vi "GenerateAnalogWaveformPiezoTraj - ZPiezo_FeedGalvo.vi"(8 "error in (no error)":errorcluster, 11 "SetupInfo_IN":T1={"ConfigParameters_Analog"={"JAI camera fps"=240.0, "Bi-Lateral Galvo xy scan range (V)"=0.7, "Bi-Lateral Galvo xy scan frequency (Hz)"=500, "AOM Blind percent (%)"=0.1, "AOM start blind percent (%) "=70.0, "ROI threshold"=1.0, "AO Sampling rate"=1000000.0}, "ConfigParameters_Digital"={"Steps per volume"=25.0, "Time per volume (s)"=0.4, "OG start layer"=15.0, "Objective Lin Rising Vel (micron/ms）"=1.0, "Image depth (micron)"=200.0, "OG latency (s)"=10.0, "OG repitation"=3.0, "OG end layer"=17.0, "Shock1 duration (s)"=0.001, "Shock2 duration (s)"=0.001, "Shock3 duration (s)"=0.01, "Shock4 duration (s)"=0.01, "Shock5 duration (s)"=0.1, "Shock duration_New"=[]}, "ConfigParameters_Other1"={"Frontal Galvo xy scan range (V)"=0.14, "Frontal Galvo xy scan frequency (Hz)"=500, "PFI 0 digital clock frequency"=500000.0, "Window size for layer index"=0.5, "sCMOS fps"=95.0}, "ConfigParameters_Others2"={"#Trials baseline"=6, "#Trials test"=6, "Time before acq. (s)"=360.0, "Time before test (s)"=600.0, "#Blocks acquisition"=5, "Inter-trial interval baseline (s)"=60.0, "#Trials per acquition block"=6, "Inter-block interval acquisition (s)"=360.0, "Inter-trial interval acquisition (s)"=20.0, "Flash latency (s)"=10.0, "Flash duration (s)"=3.2, "Response duration (s)"=10.0, "MaxTimeEventDetection (s)"=6, "StimType"=enum."Flash", "#MaxEvents"=6}, "ProcessParametersOut"={"stand Z vol Acquisition time (s)"=0.2631578947368421, "stand Z vol Backward time (s)"=0.13684210526315793, "Objective scan volt"=5.0, "Bi-lateral Galvo Z scan volt"=0.1800000180000018, "Frontal Galvo Z scan volt"=0.14940000509752818, "Objective step length (micron)"=8.0, "OG Z volet Linear Dec time (s)"=0.024, "OG Z vol Stim. steps time (s)"=0.031578947368421054, "OG Z vol Linear Acc time (s)"=0.112, "#Vol. of flash"=8, "#Vol. of shock"=1, "#Vol. bef flash"=25, "#Vol. aft flash"=17, "OG Z vol Linear Dec time (s)"=0.112, "OG Z vol time (s)"=0.39073684210526316, "Stack duration"=[0.001, 0.001, 0.01, 0.01, 0.1], "AOM stand. value size"=400000, "Plane indexing length"=0, "#Vol. blank"=0, "#Vol. blank before acq"=0, "#Vol. blank before test"=0, " #Inter-block interval acquisition (Ed-St Vol)"=0}, "WaveformParameters"={"stand Z vol Acquisition samp info"={"Fs"=1000000.0, "#s"=263158.0}, "stand Z vol Backward samp info"={"Fs"=1000000.0, "#s"=136842.0}, "OG Z vol Linear Acc samp info"={"Fs"=1000000.0, "#s"=112000.0}, "OG Z vol Stim. steps samp info"={"Fs"=1000000.0, "#s"=31579.0}, "OG Z volet Linear Dec samp info"={"Fs"=1000000.0, "#s"=24000.0}, "OG Z vol Linear Dec samp info"={"Fs"=1000000.0, "#s"=112000.0}, "OG Z vol samp info"={"Fs"=1000000.0, "#s"=390737.0}, "stand Z vol backforth samp info"={"Fs"=1000000.0, "#s"=400000.0}}, "AnalogWaveform"={"Bi-lateral Galvo Z stand waveform"={"t0"=timestamp(0 s since 1904-01-01), "dt"=1.0, "Y"=[]}, "Frontal Galvo Z stand waveform"={"t0"=timestamp(0 s since 1904-01-01), "dt"=1.0, "Y"=[]}, "Bi-lateral Galvo XY stand waveform"={"t0"=timestamp(0 s since 1904-01-01), "dt"=1.0, "Y"=[]}, "Frontal Galvo XY stand waveform"={"t0"=timestamp(0 s since 1904-01-01), "dt"=1.0, "Y"=[]}, "sCMOS stand waveform"={"t0"=timestamp(0 s since 1904-01-01), "dt"=1.0, "Y"=[]}, "Detection objective stand waveform"={"t0"=timestamp(0 s since 1904-01-01), "dt"=1.0, "Y"=[]}, "AOM stand waveform"={"t0"=timestamp(0 s since 1904-01-01), "dt"=1.0, "Y"=[]}, "PFI 0 clock stand waveform"={"t0"=timestamp(0 s since 1904-01-01), "dt"=1.0, "Y"=[]}, "Bi-lateral Galvo Z OG waveform"={"t0"=timestamp(0 s since 1904-01-01), "dt"=1.0, "Y"=[]}, "Bi-lateral Galvo XY OG waveform"={"t0"=timestamp(0 s since 1904-01-01), "dt"=1.0, "Y"=[]}, "Frontal Galvo Z OG waveform"={"t0"=timestamp(0 s since 1904-01-01), "dt"=1.0, "Y"=[]}, "Frontal Galvo XY OG waveform"={"t0"=timestamp(0 s since 1904-01-01), "dt"=1.0, "Y"=[]}, "sCMOS OG waveform"={"t0"=timestamp(0 s since 1904-01-01), "dt"=1.0, "Y"=[]}, "Detection objective OG waveform"={"t0"=timestamp(0 s since 1904-01-01), "dt"=1.0, "Y"=[]}, "AOM OG waveform"={"t0"=timestamp(0 s since 1904-01-01), "dt"=1.0, "Y"=[]}, "PFI 0 clock OG wavee"={"t0"=timestamp(0 s since 1904-01-01), "dt"=1.0, "Y"=[]}, "sCMOS blank waveform"={"t0"=timestamp(0 s since 1904-01-01), "dt"=1.0, "Y"=[]}, "All analog OG wave"=[], "All analog stand wave"=[], "All analog blank wave"=[], "BufferWaveform_Analog"=[], "Bi-lateral Galvo Z XY"={"t0"=timestamp(0 s since 1904-01-01), "dt"=1.0, "Y"=[]}, "Frontal Galvo Z XY"={"t0"=timestamp(0 s since 1904-01-01), "dt"=1.0, "Y"=[]}, "sCMOS Trigger XY"={"t0"=timestamp(0 s since 1904-01-01), "dt"=1.0, "Y"=[]}, "Detection objective XY"={"t0"=timestamp(0 s since 1904-01-01), "dt"=1.0, "Y"=[]}, "AOM XY"={"t0"=timestamp(0 s since 1904-01-01), "dt"=1.0, "Y"=[]}, "Analog_XY"=[]}, "DigitalWaveform"={"AllDigitalStandWave"=[], "AllDigialEvokedWave"=[], "AllDigialOGWave"=[], "AllDigitalPairWave_1"=[], "AllDigitalPairWave_2"=[], "AllDigitalPairWave_3"=[], "AllDigitalPairWave_4"=[], "AllDigitalPairWave_5"=[], "Plane Indexing"={"t0"=timestamp(0 s since 1904-01-01), "dt"=0.0, "Y"={"transitions"=[], "data"=[]}, "error"={"status"=FALSE, "code"=37421928, "source"=""}}, "Plane indexing P0.5 OG"={"t0"=timestamp(0 s since 1904-01-01), "dt"=0.0, "Y"={"transitions"=[], "data"=[]}, "error"={"status"=FALSE, "code"=37421928, "source"=""}}, "AllDigitalPairWaves"=[], "BufferWaveform_Digital"=[], "AllDigitalBlankWave"=[], "Digial_XY"=[]}, "PhysicalResource"={"PhysicalChannels_AI"="", "PhysicalChannels_AO"="", "PhysicalChannels_DO"="", "Task_AnalogOutput"="", "Task_DigitalOutput"="", "Task_AnalogInput"=""}, "ControlsRef"={"Mode_1"=refnum, "EventDetectionMode"=refnum, "Mode_2A"=refnum, "StimulationMode"=refnum, "Mode_2B"=refnum, "ErrorMeg"=refnum}} {"ConfigParameters_Other1"."Frontal Galvo xy scan frequency (Hz)" min=500 max=500; "ConfigParameters_Other1"."Frontal Galvo xy scan range (V)" min=0.0 max=1.5; "ConfigParameters_Analog"."AOM start blind percent (%)" min=10.0 max=90.0; "ConfigParameters_Analog"."AOM Blind percent (%)" min=0.1 max=100.0; "ConfigParameters_Analog"."Bi-Lateral Galvo xy scan frequency (Hz)" min=500 max=500; "ConfigParameters_Analog"."Bi-Lateral Galvo xy scan range (V)" min=0.0 max=1.5}) -> (0 "error out":errorcluster, 3 "SetupInfo_OUT":T1={"ConfigParameters_Analog"={"JAI camera fps"=240.0, "Bi-Lateral Galvo xy scan range (V)"=0.7, "Bi-Lateral Galvo xy scan frequency (Hz)"=500, "AOM Blind percent (%)"=0.1, "AOM start blind percent (%) "=70.0, "ROI threshold"=1.0, "AO Sampling rate"=1000000.0}, "ConfigParameters_Digital"={"Steps per volume"=25.0, "Time per volume (s)"=0.4, "OG start layer"=15.0, "Objective Lin Rising Vel (micron/ms）"=1.0, "Image depth (micron)"=200.0, "OG latency (s)"=10.0, "OG repitation"=3.0, "OG end layer"=17.0, "Shock1 duration (s)"=0.001, "Shock2 duration (s)"=0.001, "Shock3 duration (s)"=0.01, "Shock4 duration (s)"=0.01, "Shock5 duration (s)"=0.1, "Shock duration_New"=[]}, "ConfigParameters_Other1"={"Frontal Galvo xy scan range (V)"=0.14, "Frontal Galvo xy scan frequency (Hz)"=500, "PFI 0 digital clock frequency"=500000.0, "Window size for layer index"=0.5, "sCMOS fps"=95.0}, "ConfigParameters_Others2"={"#Trials baseline"=6, "#Trials test"=6, "Time before acq. (s)"=360.0, "Time before test (s)"=600.0, "#Blocks acquisition"=5, "Inter-trial interval baseline (s)"=60.0, "#Trials per acquition block"=6, "Inter-block interval acquisition (s)"=360.0, "Inter-trial interval acquisition (s)"=20.0, "Flash latency (s)"=10.0, "Flash duration (s)"=3.2, "Response duration (s)"=10.0, "MaxTimeEventDetection (s)"=6, "StimType"=enum."Flash", "#MaxEvents"=6}, "ProcessParametersOut"={"stand Z vol Acquisition time (s)"=0.2631578947368421, "stand Z vol Backward time (s)"=0.13684210526315793, "Objective scan volt"=5.0, "Bi-lateral Galvo Z scan volt"=0.1800000180000018, "Frontal Galvo Z scan volt"=0.14940000509752818, "Objective step length (micron)"=8.0, "OG Z volet Linear Dec time (s)"=0.024, "OG Z vol Stim. steps time (s)"=0.031578947368421054, "OG Z vol Linear Acc time (s)"=0.112, "#Vol. of flash"=8, "#Vol. of shock"=1, "#Vol. bef flash"=25, "#Vol. aft flash"=17, "OG Z vol Linear Dec time (s)"=0.112, "OG Z vol time (s)"=0.39073684210526316, "Stack duration"=[0.001, 0.001, 0.01, 0.01, 0.1], "AOM stand. value size"=400000, "Plane indexing length"=0, "#Vol. blank"=0, "#Vol. blank before acq"=0, "#Vol. blank before test"=0, " #Inter-block interval acquisition (Ed-St Vol)"=0}, "WaveformParameters"={"stand Z vol Acquisition samp info"={"Fs"=1000000.0, "#s"=263158.0}, "stand Z vol Backward samp info"={"Fs"=1000000.0, "#s"=136842.0}, "OG Z vol Linear Acc samp info"={"Fs"=1000000.0, "#s"=112000.0}, "OG Z vol Stim. steps samp info"={"Fs"=1000000.0, "#s"=31579.0}, "OG Z volet Linear Dec samp info"={"Fs"=1000000.0, "#s"=24000.0}, "OG Z vol Linear Dec samp info"={"Fs"=1000000.0, "#s"=112000.0}, "OG Z vol samp info"={"Fs"=1000000.0, "#s"=390737.0}, "stand Z vol backforth samp info"={"Fs"=1000000.0, "#s"=400000.0}}, "AnalogWaveform"={"Bi-lateral Galvo Z stand waveform"={"t0"=timestamp(0 s since 1904-01-01), "dt"=1.0, "Y"=[]}, "Frontal Galvo Z stand waveform"={"t0"=timestamp(0 s since 1904-01-01), "dt"=1.0, "Y"=[]}, "Bi-lateral Galvo XY stand waveform"={"t0"=timestamp(0 s since 1904-01-01), "dt"=1.0, "Y"=[]}, "Frontal Galvo XY stand waveform"={"t0"=timestamp(0 s since 1904-01-01), "dt"=1.0, "Y"=[]}, "sCMOS stand waveform"={"t0"=timestamp(0 s since 1904-01-01), "dt"=1.0, "Y"=[]}, "Detection objective stand waveform"={"t0"=timestamp(0 s since 1904-01-01), "dt"=1.0, "Y"=[]}, "AOM stand waveform"={"t0"=timestamp(0 s since 1904-01-01), "dt"=1.0, "Y"=[]}, "PFI 0 clock stand waveform"={"t0"=timestamp(0 s since 1904-01-01), "dt"=1.0, "Y"=[]}, "Bi-lateral Galvo Z OG waveform"={"t0"=timestamp(0 s since 1904-01-01), "dt"=1.0, "Y"=[]}, "Bi-lateral Galvo XY OG waveform"={"t0"=timestamp(0 s since 1904-01-01), "dt"=1.0, "Y"=[]}, "Frontal Galvo Z OG waveform"={"t0"=timestamp(0 s since 1904-01-01), "dt"=1.0, "Y"=[]}, "Frontal Galvo XY OG waveform"={"t0"=timestamp(0 s since 1904-01-01), "dt"=1.0, "Y"=[]}, "sCMOS OG waveform"={"t0"=timestamp(0 s since 1904-01-01), "dt"=1.0, "Y"=[]}, "Detection objective OG waveform"={"t0"=timestamp(0 s since 1904-01-01), "dt"=1.0, "Y"=[]}, "AOM OG waveform"={"t0"=timestamp(0 s since 1904-01-01), "dt"=1.0, "Y"=[]}, "PFI 0 clock OG wavee"={"t0"=timestamp(0 s since 1904-01-01), "dt"=1.0, "Y"=[]}, "sCMOS blank waveform"={"t0"=timestamp(0 s since 1904-01-01), "dt"=1.0, "Y"=[]}, "All analog OG wave"=[], "All analog stand wave"=[], "All analog blank wave"=[], "BufferWaveform_Analog"=[], "Bi-lateral Galvo Z XY"={"t0"=timestamp(0 s since 1904-01-01), "dt"=1.0, "Y"=[]}, "Frontal Galvo Z XY"={"t0"=timestamp(0 s since 1904-01-01), "dt"=1.0, "Y"=[]}, "sCMOS Trigger XY"={"t0"=timestamp(0 s since 1904-01-01), "dt"=1.0, "Y"=[]}, "Detection objective XY"={"t0"=timestamp(0 s since 1904-01-01), "dt"=1.0, "Y"=[]}, "AOM XY"={"t0"=timestamp(0 s since 1904-01-01), "dt"=1.0, "Y"=[]}, "Analog_XY"=[]}, "DigitalWaveform"={"AllDigitalStandWave"=[], "AllDigialEvokedWave"=[], "AllDigialOGWave"=[], "AllDigitalPairWave_1"=[], "AllDigitalPairWave_2"=[], "AllDigitalPairWave_3"=[], "AllDigitalPairWave_4"=[], "AllDigitalPairWave_5"=[], "Plane Indexing"={"t0"=timestamp(0 s since 1904-01-01), "dt"=0.0, "Y"={"transitions"=[], "data"=[]}, "error"={"status"=FALSE, "code"=37421928, "source"=""}}, "Plane indexing P0.5 OG"={"t0"=timestamp(0 s since 1904-01-01), "dt"=0.0, "Y"={"transitions"=[], "data"=[]}, "error"={"status"=FALSE, "code"=37421928, "source"=""}}, "AllDigitalPairWaves"=[], "BufferWaveform_Digital"=[], "AllDigitalBlankWave"=[], "Digial_XY"=[]}, "PhysicalResource"={"PhysicalChannels_AI"="", "PhysicalChannels_AO"="", "PhysicalChannels_DO"="", "Task_AnalogOutput"="", "Task_DigitalOutput"="", "Task_AnalogInput"=""}, "ControlsRef"={"Mode_1"=refnum, "EventDetectionMode"=refnum, "Mode_2A"=refnum, "StimulationMode"=refnum, "Mode_2B"=refnum, "ErrorMeg"=refnum}} {"ConfigParameters_Other1"."Frontal Galvo xy scan frequency (Hz)" min=500 max=500; "ConfigParameters_Other1"."Frontal Galvo xy scan range (V)" min=0.0 max=1.5; "ConfigParameters_Analog"."AOM start blind percent (%)" min=10.0 max=90.0; "ConfigParameters_Analog"."AOM Blind percent (%)" min=0.1 max=100.0; "ConfigParameters_Analog"."Bi-Lateral Galvo xy scan frequency (Hz)" min=500 max=500; "ConfigParameters_Analog"."Bi-Lateral Galvo xy scan range (V)" min=0.0 max=1.5})   [LabVIEW 2018]
uses:
  SetupInfo.ctl
  ConfigParameters_Analog.ctl
  ConfigParameters_Digital.ctl
  ConfigParameters_Others1.ctl
  ConfigParameters_Others2.ctl
  ProcessParametersOut.ctl
  WaveformParameters.ctl
  AnalogWaveform.ctl
  DigitalWaveform.ctl
  PhysicalResource.ctl
  ControlsRef.ctl
  <vilib>/Waveform/WDTOps.llb/WDT Append Waveforms DBL.vi
  <vilib>/measure/NI_MABase.lvlib
panel:
  in  "FileSamplingRate":dbl=1000.0
  in  "PiezoTrajectoryPath":path=path "D:/APP/LightSheetController_Ver8 obl/VISource/Waveform/piezo_In_Out.txt"
  out "AOM stand. value size":i32=400000
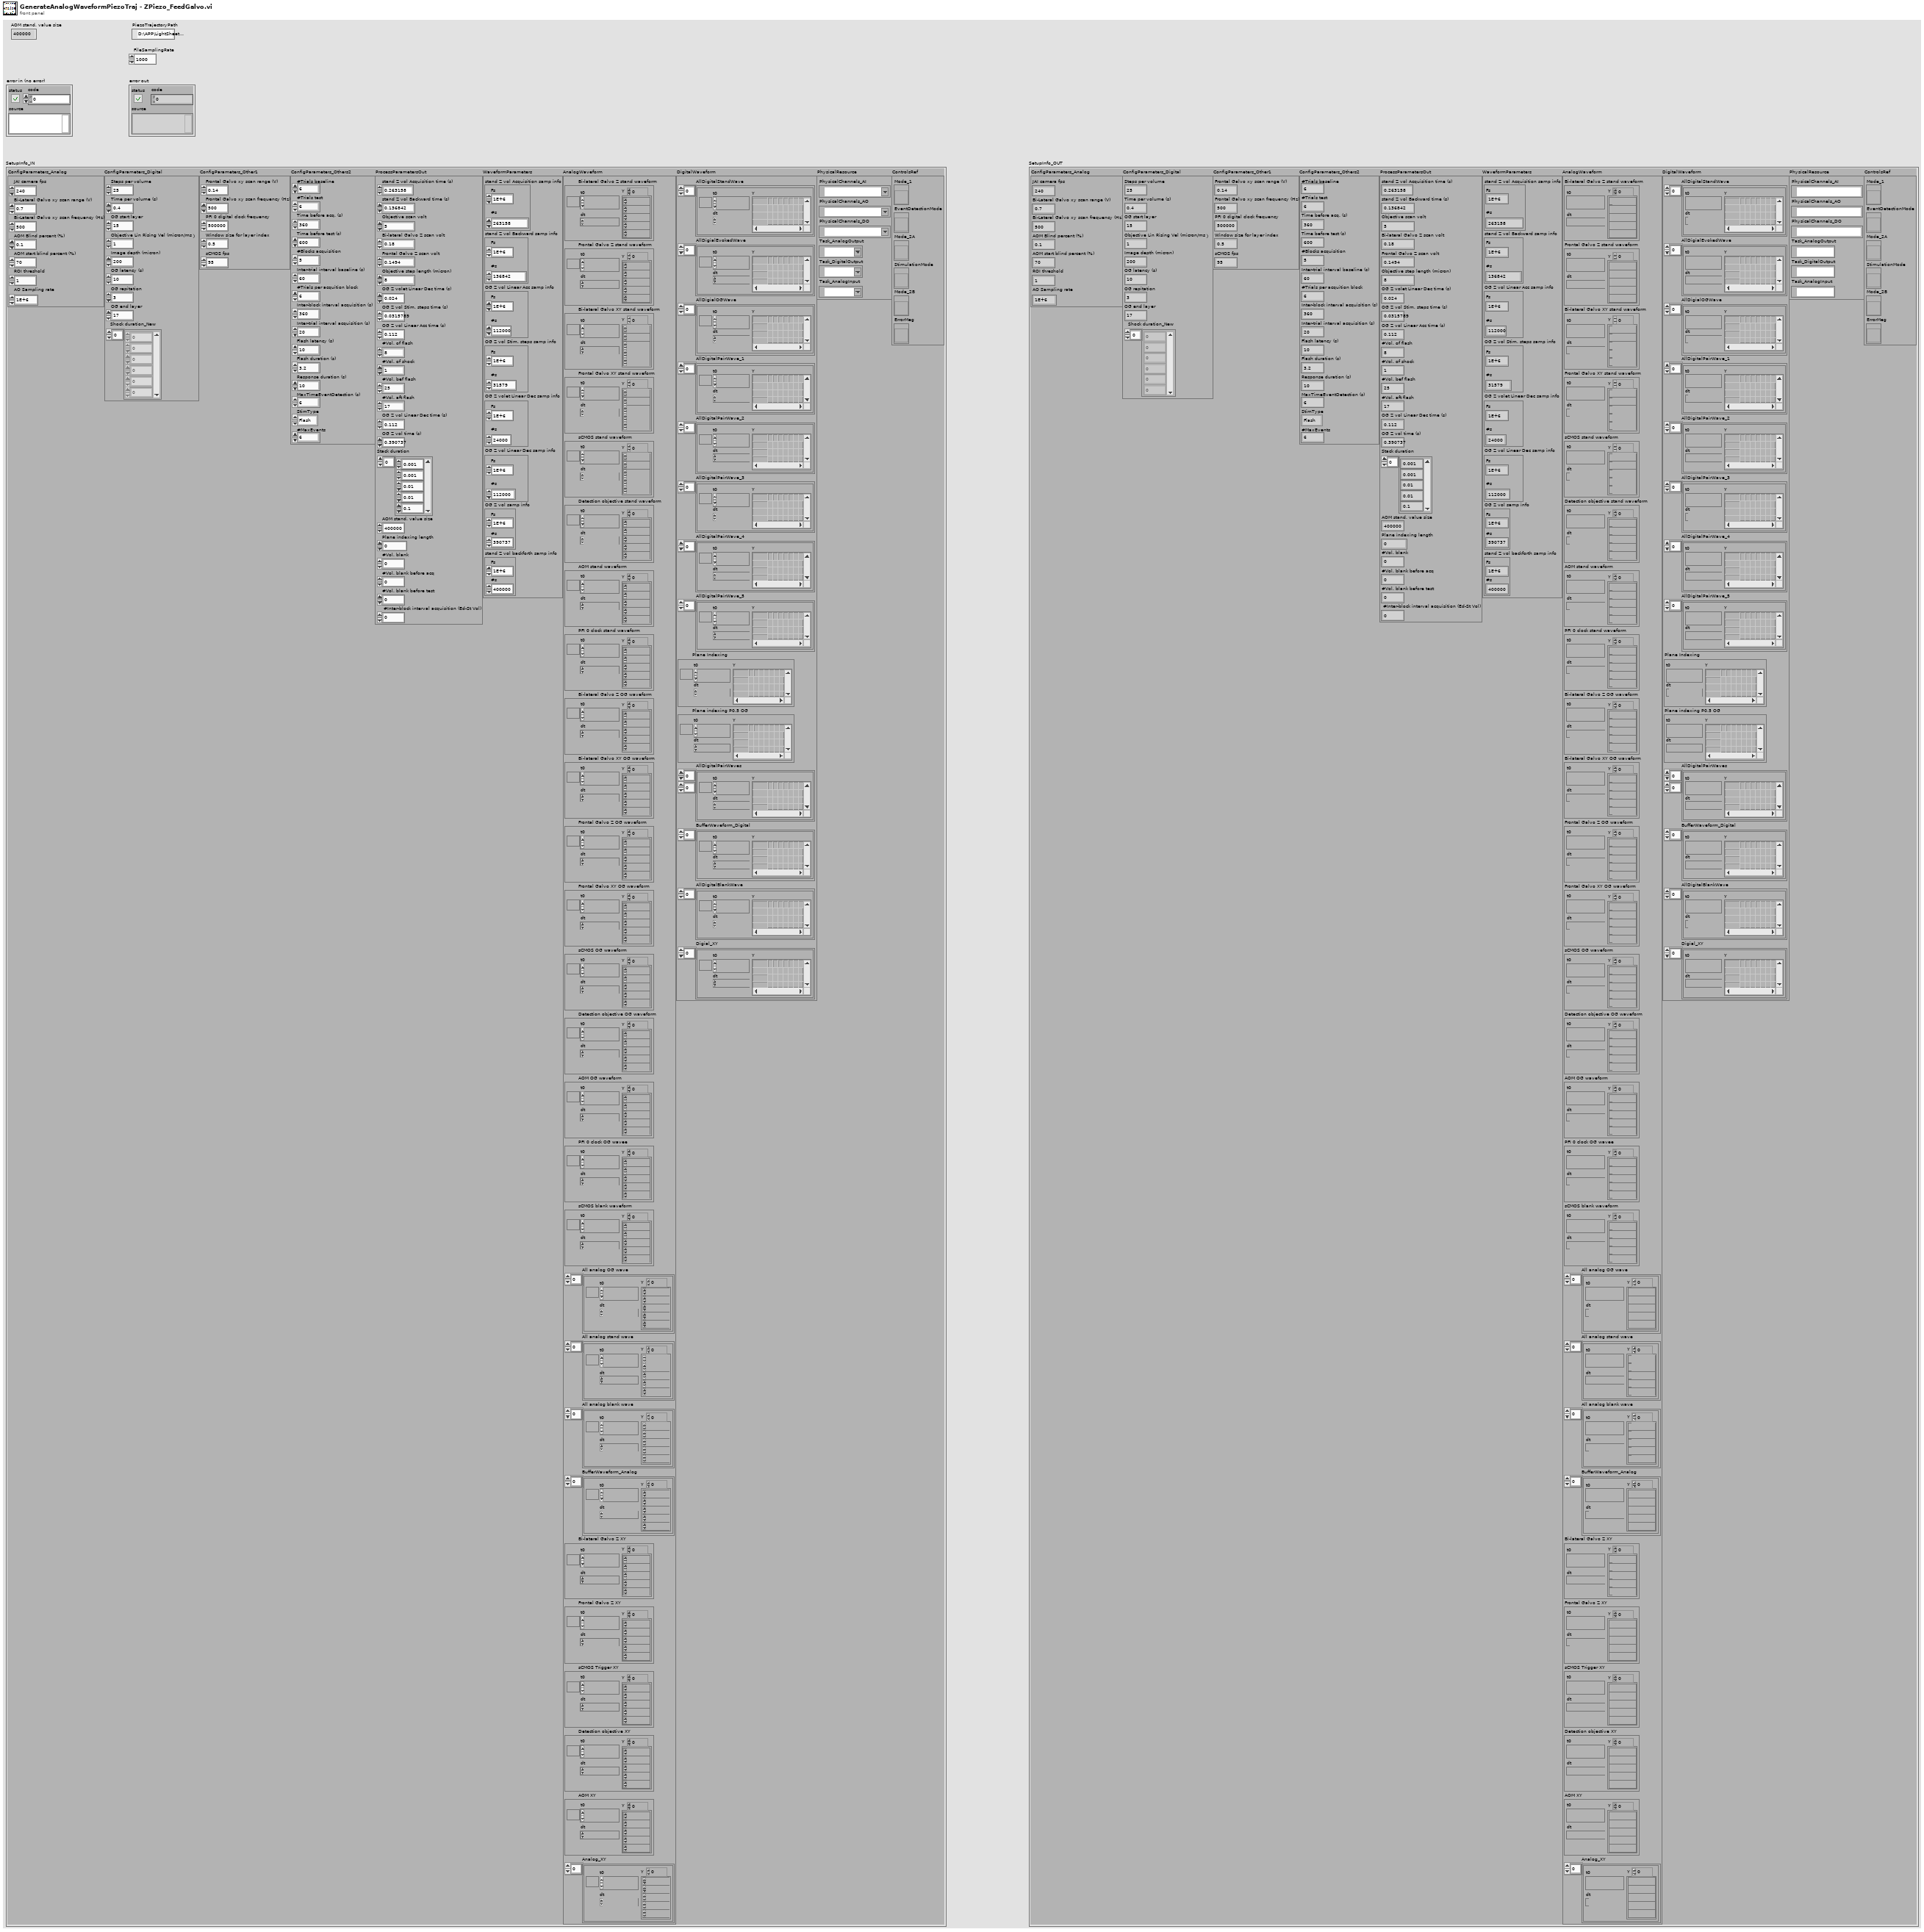
[diagram p1: front panel]
types:
  T1 = typedef "SetupInfo.ctl" = cluster{"ConfigParameters_Analog":T2, "ConfigParameters_Digital":T3, "ConfigParameters_Other1":T4, "ConfigParameters_Others2":T5, "ProcessParametersOut":T6, "WaveformParameters":T7, "AnalogWaveform":T8, "DigitalWaveform":T9, "PhysicalResource":T10, "ControlsRef":T11}
  T2 = typedef "ConfigParameters_Analog.ctl" = cluster{"JAI camera fps":dbl, "Bi-Lateral Galvo xy scan range (V)":dbl, "Bi-Lateral Galvo xy scan frequency (Hz)":i16, "AOM Blind percent (%)":dbl, "AOM start blind percent (%) ":dbl, "ROI threshold":dbl, "AO Sampling rate":dbl}
  T3 = typedef "ConfigParameters_Digital.ctl" = cluster{"Steps per volume":dbl, "Time per volume (s)":dbl, "OG start layer":dbl, "Objective Lin Rising Vel (micron/ms）":dbl, "Image depth (micron)":dbl, "OG latency (s)":dbl, "OG repitation":dbl, "OG end layer":dbl, "Shock1 duration (s)":dbl, "Shock2 duration (s)":dbl, "Shock3 duration (s)":dbl, "Shock4 duration (s)":dbl, "Shock5 duration (s)":dbl, "Shock duration_New":dbl[]}
  T4 = typedef "ConfigParameters_Others1.ctl" = cluster{"Frontal Galvo xy scan range (V)":dbl, "Frontal Galvo xy scan frequency (Hz)":i16, "PFI 0 digital clock frequency":dbl, "Window size for layer index":dbl, "sCMOS fps":dbl}
  T5 = typedef "ConfigParameters_Others2.ctl" = cluster{"#Trials baseline":i32, "#Trials test":i32, "Time before acq. (s)":dbl, "Time before test (s)":dbl, "#Blocks acquisition":i32, "Inter-trial interval baseline (s)":dbl, "#Trials per acquition block":i32, "Inter-block interval acquisition (s)":dbl, "Inter-trial interval acquisition (s)":dbl, "Flash latency (s)":dbl, "Flash duration (s)":dbl, "Response duration (s)":dbl, "MaxTimeEventDetection (s)":i32, "StimType":enum16{"Flash", "OG"}, "#MaxEvents":i32}
  T6 = typedef "ProcessParametersOut.ctl" = cluster{"stand Z vol Acquisition time (s)":dbl, "stand Z vol Backward time (s)":dbl, "Objective scan volt":dbl, "Bi-lateral Galvo Z scan volt":dbl, "Frontal Galvo Z scan volt":dbl, "Objective step length (micron)":dbl, "OG Z volet Linear Dec time (s)":dbl, "OG Z vol Stim. steps time (s)":dbl, "OG Z vol Linear Acc time (s)":dbl, "#Vol. of flash":i32, "#Vol. of shock":i32, "#Vol. bef flash":i32, "#Vol. aft flash":i32, "OG Z vol Linear Dec time (s)":dbl, "OG Z vol time (s)":dbl, "Stack duration":dbl[], "AOM stand. value size":i32, "Plane indexing length":i32, "#Vol. blank":i32, "#Vol. blank before acq":i32, "#Vol. blank before test":i32, " #Inter-block interval acquisition (Ed-St Vol)":i32}
  T7 = typedef "WaveformParameters.ctl" = cluster{"stand Z vol Acquisition samp info":cluster{"Fs":dbl, "#s":dbl}, "stand Z vol Backward samp info":cluster{"Fs":dbl, "#s":dbl}, "OG Z vol Linear Acc samp info":cluster{"Fs":dbl, "#s":dbl}, "OG Z vol Stim. steps samp info":cluster{"Fs":dbl, "#s":dbl}, "OG Z volet Linear Dec samp info":cluster{"Fs":dbl, "#s":dbl}, "OG Z vol Linear Dec samp info":cluster{"Fs":dbl, "#s":dbl}, "OG Z vol samp info":cluster{"Fs":dbl, "#s":dbl}, "stand Z vol backforth samp info":cluster{"Fs":dbl, "#s":dbl}}
  T8 = typedef "AnalogWaveform.ctl" = cluster{"Bi-lateral Galvo Z stand waveform":waveform(dbl), "Frontal Galvo Z stand waveform":waveform(dbl), "Bi-lateral Galvo XY stand waveform":waveform(dbl), "Frontal Galvo XY stand waveform":waveform(dbl), "sCMOS stand waveform":waveform(dbl), "Detection objective stand waveform":waveform(dbl), "AOM stand waveform":waveform(dbl), "PFI 0 clock stand waveform":waveform(dbl), "Bi-lateral Galvo Z OG waveform":waveform(dbl), "Bi-lateral Galvo XY OG waveform":waveform(dbl), "Frontal Galvo Z OG waveform":waveform(dbl), "Frontal Galvo XY OG waveform":waveform(dbl), "sCMOS OG waveform":waveform(dbl), "Detection objective OG waveform":waveform(dbl), "AOM OG waveform":waveform(dbl), "PFI 0 clock OG wavee":waveform(dbl), "sCMOS blank waveform":waveform(dbl), "All analog OG wave":waveform(dbl)[], "All analog stand wave":waveform(dbl)[], "All analog blank wave":waveform(dbl)[], "BufferWaveform_Analog":waveform(dbl)[], "Bi-lateral Galvo Z XY":waveform(dbl), "Frontal Galvo Z XY":waveform(dbl), "sCMOS Trigger XY":waveform(dbl), "Detection objective XY":waveform(dbl), "AOM XY":waveform(dbl), "Analog_XY":waveform(dbl)[]}
  T9 = typedef "DigitalWaveform.ctl" = cluster{"AllDigitalStandWave":digitalwaveform[], "AllDigialEvokedWave":digitalwaveform[], "AllDigialOGWave":digitalwaveform[], "AllDigitalPairWave_1":digitalwaveform[], "AllDigitalPairWave_2":digitalwaveform[], "AllDigitalPairWave_3":digitalwaveform[], "AllDigitalPairWave_4":digitalwaveform[], "AllDigitalPairWave_5":digitalwaveform[], "Plane Indexing":digitalwaveform, "Plane indexing P0.5 OG":digitalwaveform, "AllDigitalPairWaves":digitalwaveform[][], "BufferWaveform_Digital":digitalwaveform[], "AllDigitalBlankWave":digitalwaveform[], "Digial_XY":digitalwaveform[]}
  T10 = typedef "PhysicalResource.ctl" = cluster{"PhysicalChannels_AI":tag, "PhysicalChannels_AO":tag, "PhysicalChannels_DO":tag, "Task_AnalogOutput":refnum<k21>, "Task_DigitalOutput":refnum<k21>, "Task_AnalogInput":refnum<k21>}
  T11 = typedef "ControlsRef.ctl" = cluster{"Mode_1":refnum<vi>, "EventDetectionMode":refnum<vi>, "Mode_2A":refnum<vi>, "StimulationMode":refnum<vi>, "Mode_2B":refnum<vi>, "ErrorMeg":refnum<vi>}
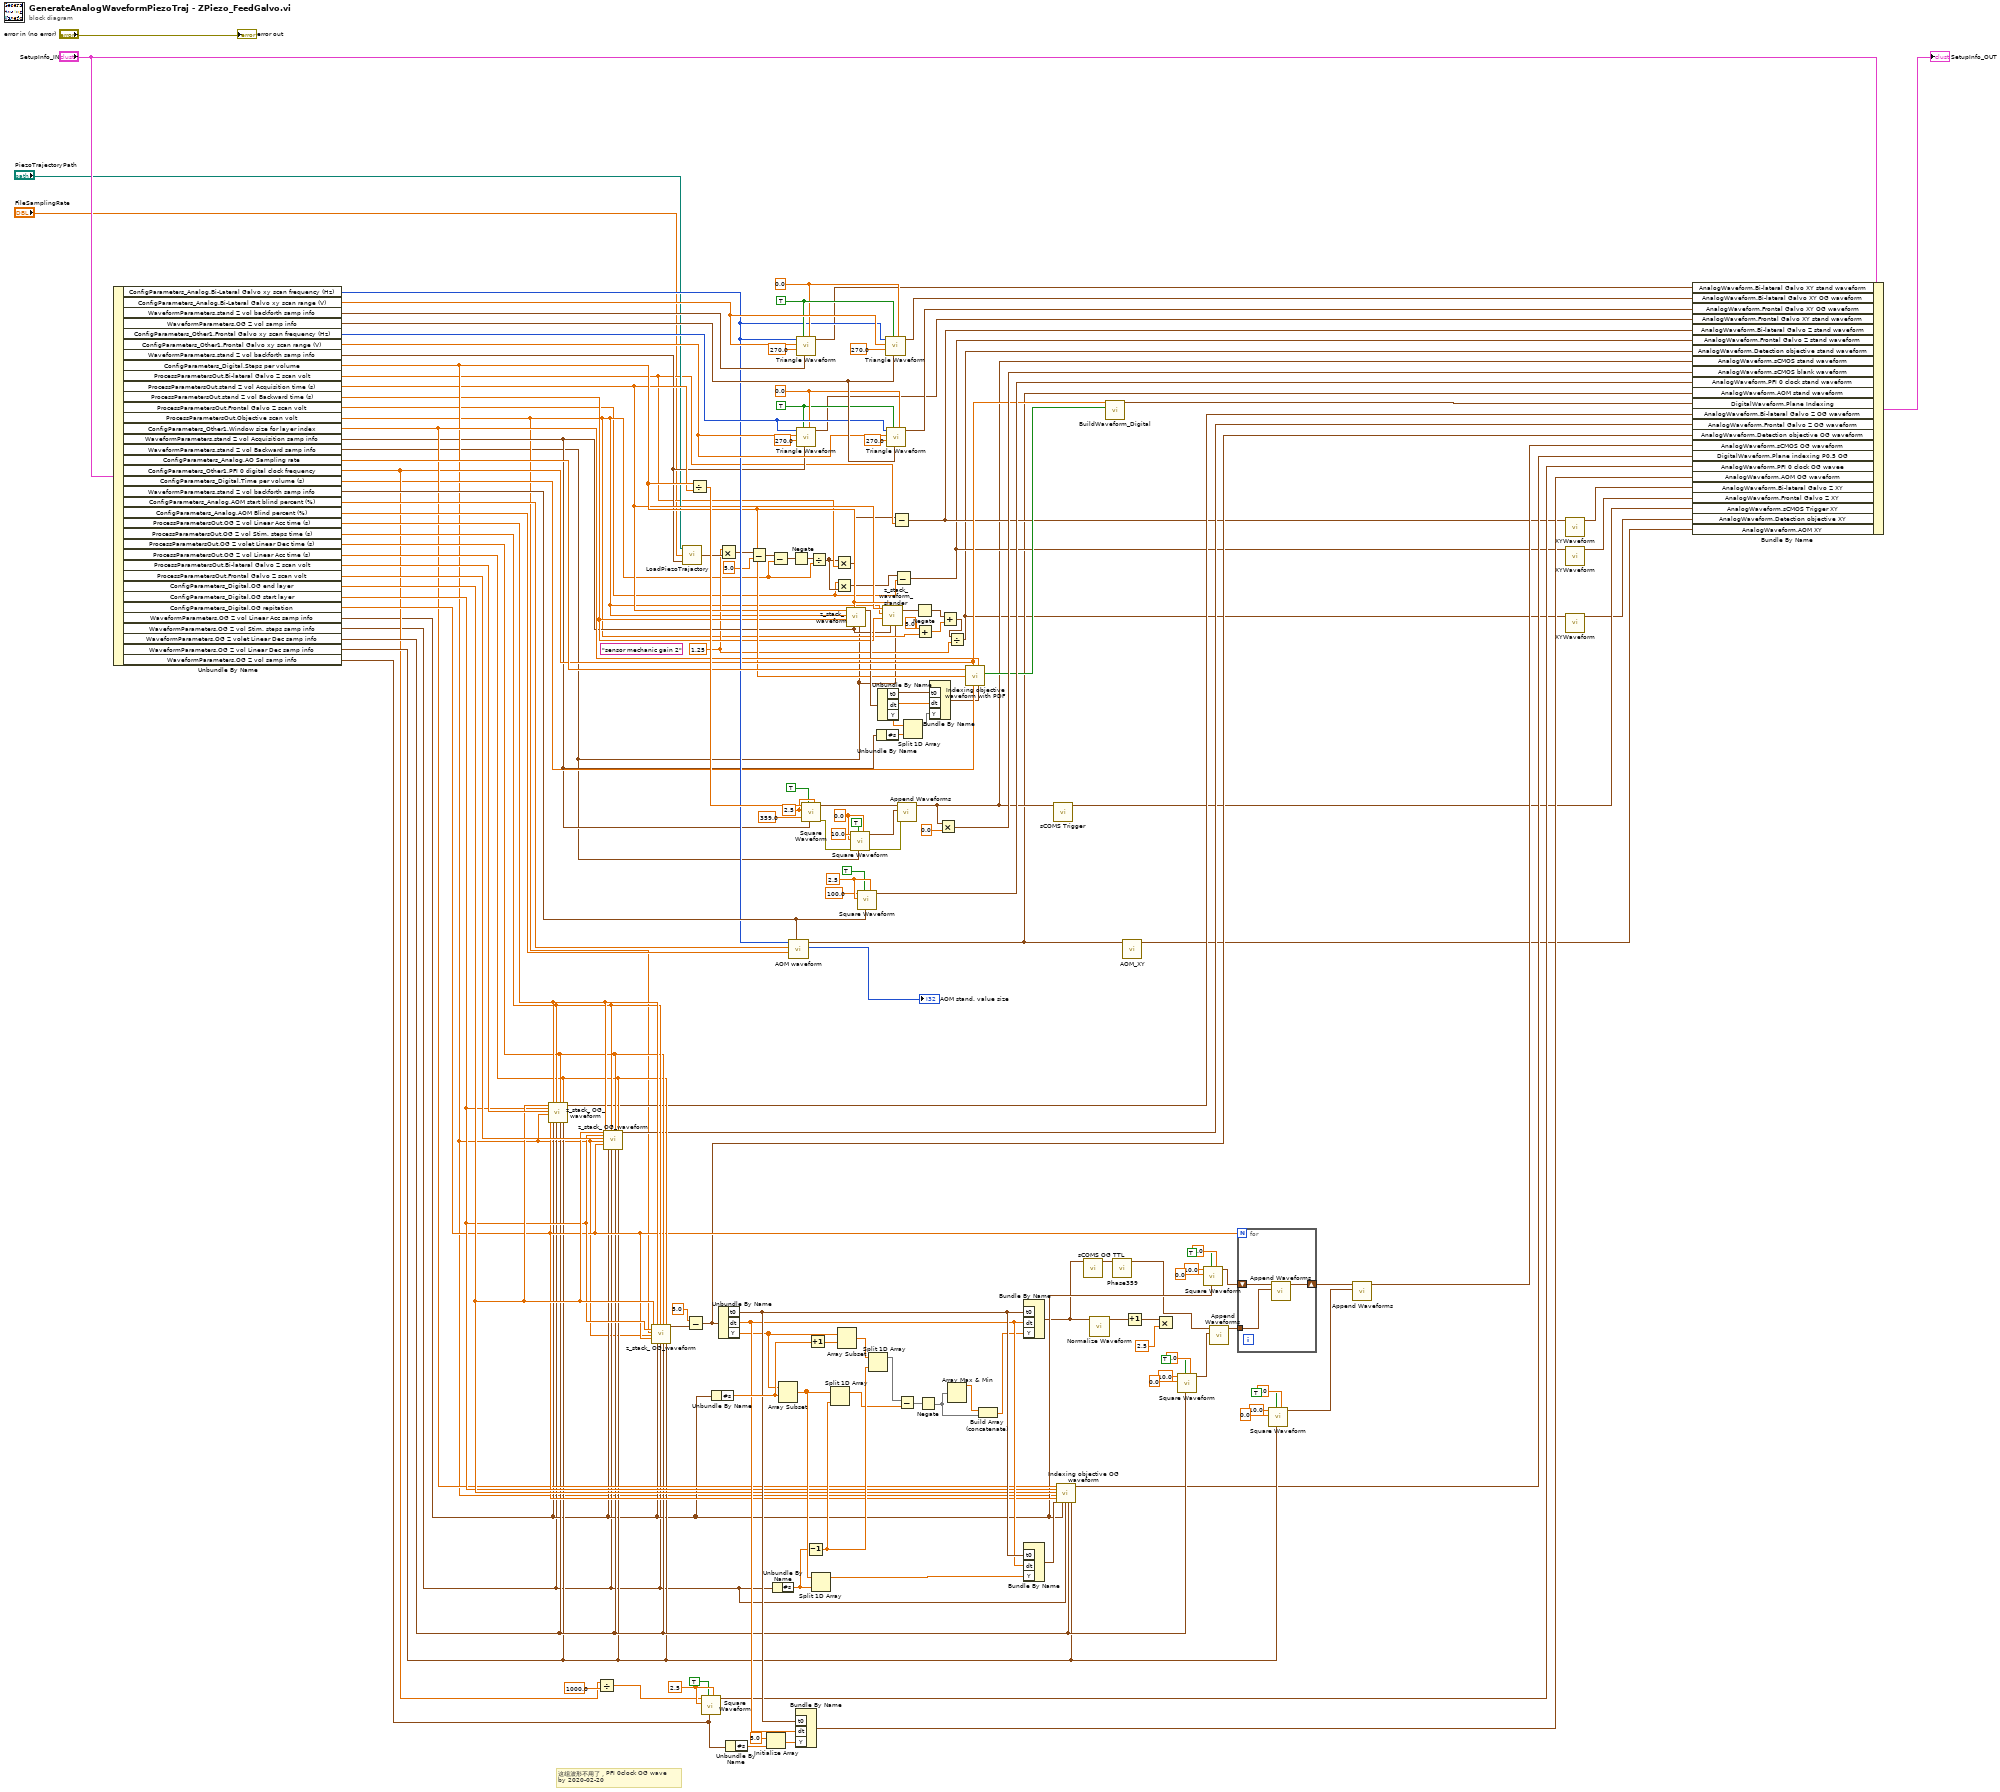
[diagram p0: block diagram]
diagram:
  (unwired) "sensor mechanic gain 2"
  w15 = 1.25
  w91 = 2.5
  w136 = 2.5 ("offset")
  w143 = 0.0 ("offset")
  w147 = 2.5 ("amplitude")
  w122 = TRUE ("reset signal")
  w130 = TRUE ("reset signal")
  w129 = 0.0 ("offset")
  w123 = 0.0 ("offset")
  # "这组波形不用了，PFI 0clock OG wave\nby 2020-02-20"
  n1 = Unbundle By Name("SetupInfo_IN") -> ("ConfigParameters_Analog.Bi-Lateral Galvo xy scan frequency (Hz)"=w118:i16, "ConfigParameters_Analog.Bi-Lateral Galvo xy scan range (V)"=w132:dbl, "WaveformParameters.stand Z vol backforth samp info"=w131:cluster{"Fs":dbl, "#s":dbl}, "WaveformParameters.OG Z vol samp info"=w127:cluster{"Fs":dbl, "#s":dbl}, "ConfigParameters_Other1.Frontal Galvo xy scan frequency (Hz)"=w126:i16, "ConfigParameters_Other1.Frontal Galvo xy scan range (V)"=w125:dbl, "WaveformParameters.stand Z vol backforth samp info"=w18:cluster{"Fs":dbl, "#s":dbl}, "ConfigParameters_Digital.Steps per volume"=w24:dbl, "ProcessParametersOut.Bi-lateral Galvo Z scan volt"=w7:dbl, "ProcessParametersOut.stand Z vol Acquisition time (s)"=w23:dbl, "ProcessParametersOut.stand Z vol Backward time (s)"=w22:dbl, "ProcessParametersOut.Frontal Galvo Z scan volt"=w4:dbl, "ProcessParametersOut.Objective scan volt"=w8:dbl, "ConfigParameters_Other1.Window size for layer index"=w75:dbl, "WaveformParameters.stand Z vol Acquisition samp info"=w21:cluster{"Fs":dbl, "#s":dbl}, "WaveformParameters.stand Z vol Backward samp info"=w2:cluster{"Fs":dbl, "#s":dbl}, "ConfigParameters_Analog.AO Sampling rate"=w120:dbl, "ConfigParameters_Other1.PFI 0 digital clock frequency"=w59:dbl, "ConfigParameters_Digital.Time per volume (s)"=w58:dbl, "WaveformParameters.stand Z vol backforth samp info"=w119:cluster{"Fs":dbl, "#s":dbl}, "ConfigParameters_Analog.AOM start blind percent (%)"=w117:dbl, "ConfigParameters_Analog.AOM Blind percent (%)"=w116:dbl, "ProcessParametersOut.OG Z vol Linear Acc time (s)"=w84:dbl, "ProcessParametersOut.OG Z vol Stim. steps time (s)"=w83:dbl, "ProcessParametersOut.OG Z volet Linear Dec time (s)"=w82:dbl, "ProcessParametersOut.OG Z vol Linear Acc time (s)"=w81:dbl, "ProcessParametersOut.Bi-lateral Galvo Z scan volt"=w80:dbl, "ProcessParametersOut.Frontal Galvo Z scan volt"=w79:dbl, "ConfigParameters_Digital.OG end layer"=w78:dbl, "ConfigParameters_Digital.OG start layer"=w77:dbl, "ConfigParameters_Digital.OG repitation"=w76:dbl, "WaveformParameters.OG Z vol Linear Acc samp info"=w41:cluster{"Fs":dbl, "#s":dbl}, "WaveformParameters.OG Z vol Stim. steps samp info"=w40:cluster{"Fs":dbl, "#s":dbl}, "WaveformParameters.OG Z volet Linear Dec samp info"=w74:cluster{"Fs":dbl, "#s":dbl}, "WaveformParameters.OG Z vol Linear Dec samp info"=w73:cluster{"Fs":dbl, "#s":dbl}, "WaveformParameters.OG Z vol samp info"=w72:cluster{"Fs":dbl, "#s":dbl})
  n2 = call "z_stack_ OG_waveform.vi"("OG end layer"=w78, "OG start layer"=w77, "SPECIFIC scan volt"=w80, "Steps per volume"=w24, "OG repitation"=w76, "Objective线性加速时间"=w84, "OG Z stack 线性加速 采样信息"=w41, "Objective 刺激steps 时间（s）"=w83, "OG Z stack 刺激steps 采样信息"=w40, "Objective volet 线性减速 时间（s）"=w82, "OG Z volet 线性减速 采样信息"=w74, "Objective线性减速时间"=w81, "OG Z stack 线性减速 采样信息"=w73) -> ("waveform out"=w62:waveform(dbl))  [unwired: 2 in, 4 out]
  n3 = Divide(x=w59, y=1000.0) -> (x/y=w65:dbl)
  n4 = call "z_stack_ OG_waveform.vi"("OG end layer"=w78, "OG start layer"=w77, "SPECIFIC scan volt"=w79, "Steps per volume"=w24, "OG repitation"=w76, "Objective线性加速时间"=w84, "OG Z stack 线性加速 采样信息"=w41, "Objective 刺激steps 时间（s）"=w83, "OG Z stack 刺激steps 采样信息"=w40, "Objective volet 线性减速 时间（s）"=w82, "OG Z volet 线性减速 采样信息"=w74, "Objective线性减速时间"=w81, "OG Z stack 线性减速 采样信息"=w73) -> ("waveform out"=w61:waveform(dbl))  [unwired: 2 in, 4 out]
  n5 = call "z_stack_ OG_waveform.vi"("OG end layer"=w78, "OG start layer"=w77, "SPECIFIC scan volt"=w8, "Steps per volume"=w24, "OG repitation"=w76, "Objective线性加速时间"=w84, "OG Z stack 线性加速 采样信息"=w41, "Objective 刺激steps 时间（s）"=w83, "OG Z stack 刺激steps 采样信息"=w40, "Objective volet 线性减速 时间（s）"=w82, "OG Z volet 线性减速 采样信息"=w74, "Objective线性减速时间"=w81, "OG Z stack 线性减速 采样信息"=w73) -> ("waveform out"=w54:waveform(dbl))  [unwired: 2 in, 4 out]
  n6 = call "LoadPiezoTrajactory.vi"("Z backforth 采样信息"=w18, "File Sampling Rate"="FileSamplingRate", "Path"="PiezoTrajectoryPath") -> ("output waveform"=w16:waveform(dbl))
  n7 = Subtract(x=5.0, y=w54) -> (x-y=w49:waveform(dbl))
  n8 = Divide(x=w24, y=w23) -> (x/y=w148:dbl)
  n9 = call <vilib>:"Square Waveform.vi"("offset"=w91, "sampling info"=w72, "reset signal"=TRUE, "amplitude"=w91, "frequency"=w65) -> ("signal out"=w70:waveform(dbl))  [unwired: 5 in, 1 out]
  n10 = Unbundle By Name(w41) -> ("#s"=w92:dbl)
  n11 = Unbundle By Name(w49) -> ("t0"=w87:timestamp, "dt"=w86:dbl, "Y"=w52:dbl[])
  n12 = Multiply(x=w15, y=w16) -> (x*y=w14:waveform(dbl))
  n13 = Unbundle By Name(w72) -> ("#s"=w85:dbl)
  n14 = Subtract(x=w14, y=5.0) -> (x-y=w13:waveform(dbl))
  n15 = Initialize Array(5.0 ("element"), w85) -> (w88:dbl[])
  n16 = Subtract(x=w13, y=w8) -> (x-y=w10:waveform(dbl))
  n17 = Unbundle By Name(w40) -> ("#s"=w93:dbl)
  n18 = Array Subset(array=w52, index=w92) -> (w109:dbl[])  [unwired: 1 in]
  n19 = call "AOM waveform.vi"("z stack 往复采样信息"=w119, "AOM Blind percent (%)"=w116, "AOM start blind percent (%)"=w117, "Bi-Lateral Galvo xy scan frequency (Hz)"=w118) -> ("数值"=→"AOM stand. value size":i32, "Waveform"=w26:waveform(dbl))  [unwired: 6 in]
  n20 = Negate(x=w10) -> (-x=w9:waveform(dbl))
  n21 = Bundle By Name("t0"=w87, "dt"=w86, "Y"=w88) -> (w69:waveform(dbl))  [unwired: 1 in]
  n22 = call <vilib>:"Triangle Waveform.vi"("offset"=w129, "sampling info"=w131, "reset signal"=w130, "phase"=270.0, "amplitude"=w132, "frequency"=w118) -> ("signal out"=w67:waveform(dbl))  [unwired: 4 in, 1 out]
  n23 = call <vilib>:"Triangle Waveform.vi"("offset"=w123, "sampling info"=w18, "reset signal"=w122, "phase"=270.0, "amplitude"=w125, "frequency"=w126) -> ("signal out"=w121:waveform(dbl))  [unwired: 4 in, 1 out]
  n24 = call <vilib>:"Square Waveform.vi"("offset"=w147, "sampling info"=w21, "reset signal"=TRUE, "phase"=359.0, "amplitude"=w147, "frequency"=w148) -> ("error out"=w141:errorcluster, "signal out"=w139:waveform(dbl))  [unwired: 4 in]
  n25 = Decrement(x=w93) -> (x-1=w110:dbl)
  n26 = Increment(x=w92) -> (x+1=w111:dbl)
  n27 = Divide(x=w9, y=w8) -> (x/y=w5:waveform(dbl))
  n28 = Split 1D Array(array=w109, index=w93) -> (first subarray=w108:dbl[])  [unwired: 1 out]
  n29 = Split 1D Array(array=w109, index=w110) -> (first subarray=w45:dbl[])  [unwired: 1 out]
  n30 = Multiply(x=w5, y=w7) -> (x*y=w6:waveform(dbl))
  n31 = Multiply(x=w4, y=w5) -> (x*y=w3:waveform(dbl))
  n32 = Array Subset(array=w52, index=w111) -> (w51:dbl[])  [unwired: 1 in]
  n33 = call "z_stack_waveform.vi"("Z stack backward"=w2, "Z stack acquisition"=w21, "Steps per Volume"=w24, "Backward Time (s)"=w22, "SPECIFIC scan volt"=w8, "Aquisition Time (s)"=w23) -> ("WaveformOut"=w56:waveform(dbl))  [unwired: 5 in]
  n34 = call <vilib>:"Square Waveform.vi"("offset"=w143, "sampling info"=w2, "reset signal"=TRUE, "error in (no error)"=w141, "amplitude"=w143, "frequency"=10.0) -> ("error out"=w138:errorcluster, "signal out"=w140:waveform(dbl))  [unwired: 4 in]
  n35 = call <vilib>:"Square Waveform.vi"("offset"=w136, "sampling info"=w119, "reset signal"=TRUE, "amplitude"=w136, "frequency"=100.0 ("amplitude")) -> ("signal out"=w114:waveform(dbl))  [unwired: 5 in, 1 out]
  n36 = Split 1D Array(array=w51, index=w110) -> (first subarray=w46:dbl[])  [unwired: 1 out]
  n37 = Unbundle By Name(w21) -> ("#s"=w150:dbl)
  n38 = Unbundle By Name(w56) -> ("t0"=w153:timestamp, "dt"=w152:dbl, "Y"=w151:dbl[])
  n39 = call "z_stack_waveform_slander.vi"("Z stack backward"=w2, "Z stack acquisition"=w21, "Steps per Volume"=w24, "Backward Time (s)"=w22, "SPECIFIC scan volt"=w8, "Aquisition Time (s)"=w23) -> ("WaveformOut"=w25:waveform(dbl))  [unwired: 5 in]
  n40 = call <vilib>:"Triangle Waveform.vi"("offset"=w129, "sampling info"=w127, "reset signal"=w130, "phase"=270.0, "amplitude"=w132, "frequency"=w118) -> ("signal out"=w128:waveform(dbl))  [unwired: 4 in, 1 out]
  n41 = call <vilib>:"Triangle Waveform.vi"("offset"=w123, "sampling info"=w127, "reset signal"=w122, "phase"=270.0, "amplitude"=w125, "frequency"=w126) -> ("signal out"=w124:waveform(dbl))  [unwired: 4 in, 1 out]
  n42 = Subtract(x=w6, y=w7) -> (x-y=w34:waveform(dbl))
  n43 = Subtract(x=w3, y=w4) -> (x-y=w32:waveform(dbl))
  n44 = call-poly <vilib>:"Append Waveforms.vi"("error in (no error)"=w138, "waveform B"=w140, "waveform A"=w139) -> ("waveform out"=w30:waveform(dbl))  [unwired: 7 in, 1 out]
  n45 = Subtract(x=w46, y=w45) -> (x-y=w43:dbl[])
  n46 = Split 1D Array(array=w151, index=w150) -> (first subarray=w149:dbl[])  [unwired: 1 out]
  n47 = Negate(x=w25) -> (-x=w155:waveform(dbl))
  n48 = Add(x=5.0, y=w8) -> (x+y=w154:dbl)
  n49 = Negate(x=w43) -> (-x=w50:dbl[])
  n50 = Bundle By Name("t0"=w153, "dt"=w152, "Y"=w149) -> (w57:waveform(dbl))  [unwired: 1 in]
  n51 = Multiply(x=w30, y=0.0) -> (x*y=w115:waveform(dbl))
  n52 = Add(x=w155, y=w154) -> (x+y=w20:waveform(dbl))
  n53 = Divide(x=w20, y=w15) -> (x/y=w19:waveform(dbl))
  n54 = Array Max & Min(array=w50) -> (max value=w112:dbl)  [unwired: 3 out]
  n55 = call "Indexing objective waveform with PDF.vi"("AO sampling rate"=w120, "PFI0 digital clock frequency"=w59, "Steps per Volume"=w24, "Time per volume (s)"=w58, "Window size for layer index (ms)"=w75, "Steps Waveform"=w57) -> ("Plane Indexing data"=w64:bool[])  [unwired: 3 in, 1 out]
  n56 = Build Array (concatenate)(w112, w50) -> (w42:dbl[])
  n57 = Bundle By Name("t0"=w87, "dt"=w86, "Y"=w42) -> (w38:waveform(dbl))  [unwired: 1 in]
  n58 = Bundle By Name("t0"=w87, "dt"=w86, "Y"=w108) -> (w107:waveform(dbl))  [unwired: 1 in]
  n59 = call "sCOMS Trigger.vi"("In"=w30) -> ("Out"=w29:waveform(dbl))  [unwired: 10 in]
  n60 = call "Indexing objective OG waveform.vi"("Window size for layer index"=w75, "OG start layer"=w77, "OG end layer"=w78, "Steps per Volume"=w24, "OG repitation"=w76, "Waveform"=w107, "OG Z 线性加速 采样信息"=w41, "OG Z stack 刺激 steps 采样信息"=w40, "OG Z volet 线性减速 采样信息"=w74, "OG Z 线性减速 采样信息"=w73) -> ("Waveform_Digital"=w71:digitalwaveform)  [unwired: 9 in]
  n61 = call "sCOMS OG TTL.vi"("DataIn"=w38) -> ("Out"=w36:waveform(dbl))  [unwired: 10 in]
  n62 = call <vilib>:"Normalize Waveform.vi"("waveform in"=w38) -> ("normalized waveform"=w53:waveform(dbl))  [unwired: 7 in, 3 out]
  n63 = call "BuildWaveform_Digital.vi"("DigitalData"=w64, "SampleRate"=w59) -> ("DigitalWaveformOut"=w60:digitalwaveform)  [unwired: 9 in]
  n64 = call "Phase359.vi"("DataIn"=w36) -> ("DataOut"=w35:waveform(dbl))  [unwired: 10 in]
  n65 = call "AOM_XY.vi"("In"=w26) -> ("Out"=w27:waveform(dbl))  [unwired: 10 in]
  n66 = Increment(x=w53) -> (x+1=w55:waveform(dbl))
  n67 = Multiply(x=w55, y=2.5) -> ()  [unwired: 1 out]
  n68 = call <vilib>:"Square Waveform.vi"("offset"=0.0, "sampling info"=w74, "reset signal"=TRUE, "amplitude"=0.0, "frequency"=10.0) -> ("signal out"=w102:waveform(dbl))  [unwired: 5 in, 1 out]
  n69 = call <vilib>:"Square Waveform.vi"("offset"=0.0, "sampling info"=w41, "reset signal"=TRUE, "amplitude"=0.0, "frequency"=10.0) -> ("signal out"=w48:waveform(dbl))  [unwired: 5 in, 1 out]
  n70 = call-poly <vilib>:"Append Waveforms.vi"("waveform B"=w102, "waveform A"=w35) -> ("waveform out"=w47:waveform(dbl))  [unwired: 8 in, 1 out]
  n71 = for {
    N: w76 -> [_]
    tunnel: w47 -> [w164]
    shift-right: [w162] -> w39
    shift-left: w48 -> [w163]
    n72 = call-poly <vilib>:"Append Waveforms.vi"("waveform B"=w164, "waveform A"=w163) -> ("waveform out"=w162:waveform(dbl))  [unwired: 8 in, 1 out]
  }
  n73 = call <vilib>:"Square Waveform.vi"("offset"=0.0, "sampling info"=w73, "reset signal"=TRUE, "amplitude"=0.0, "frequency"=10.0) -> ("signal out"=w44:waveform(dbl))  [unwired: 5 in, 1 out]
  n74 = call-poly <vilib>:"Append Waveforms.vi"("waveform B"=w44, "waveform A"=w39) -> ("waveform out"=w37:waveform(dbl))  [unwired: 8 in, 1 out]
  n75 = call "XYWaveform.vi"("XYWaveformIN"=w34) -> ("XYWaveformOut"=w33:waveform(dbl))  [unwired: 10 in]
  n76 = call "XYWaveform.vi"("XYWaveformIN"=w32) -> ("XYWaveformOut"=w31:waveform(dbl))  [unwired: 10 in]
  n77 = call "XYWaveform.vi"("XYWaveformIN"=w19) -> ("XYWaveformOut"=w28:waveform(dbl))  [unwired: 10 in]
  n78 = Bundle By Name(cluster="SetupInfo_IN", "AnalogWaveform.Bi-lateral Galvo XY stand waveform"=w67, "AnalogWaveform.Bi-lateral Galvo XY OG waveform"=w128, "AnalogWaveform.Frontal Galvo XY OG waveform"=w124, "AnalogWaveform.Frontal Galvo XY stand waveform"=w121, "AnalogWaveform.Bi-lateral Galvo Z stand waveform"=w34, "AnalogWaveform.Frontal Galvo Z stand waveform"=w32, "AnalogWaveform.Detection objective stand waveform"=w19, "AnalogWaveform.sCMOS stand waveform"=w30, "AnalogWaveform.sCMOS blank waveform"=w115, "AnalogWaveform.PFI 0 clock stand waveform"=w114, "AnalogWaveform.AOM stand waveform"=w26, "DigitalWaveform.Plane Indexing"=w60, "AnalogWaveform.Bi-lateral Galvo Z OG waveform"=w62, "AnalogWaveform.Frontal Galvo Z OG waveform"=w61, "AnalogWaveform.Detection objective OG waveform"=w49, "AnalogWaveform.sCMOS OG waveform"=w37, "DigitalWaveform.Plane indexing P0.5 OG"=w71, "AnalogWaveform.PFI 0 clock OG wavee"=w70, "AnalogWaveform.AOM OG waveform"=w69, "AnalogWaveform.Bi-lateral Galvo Z XY"=w33, "AnalogWaveform.Frontal Galvo Z XY"=w31, "AnalogWaveform.sCMOS Trigger XY"=w29, "AnalogWaveform.Detection objective XY"=w28, "AnalogWaveform.AOM XY"=w27) -> (→"SetupInfo_OUT":T1)
  "error out" <- "error in (no error)"
